vi "3.4.vi"() -> ()   [LabVIEW 2017]
panel:
  out "长度":dbl
  in  "字符串 2":string
  in  "字符串":string
  out "结果字符串":string
  in  "输入 1":dbl
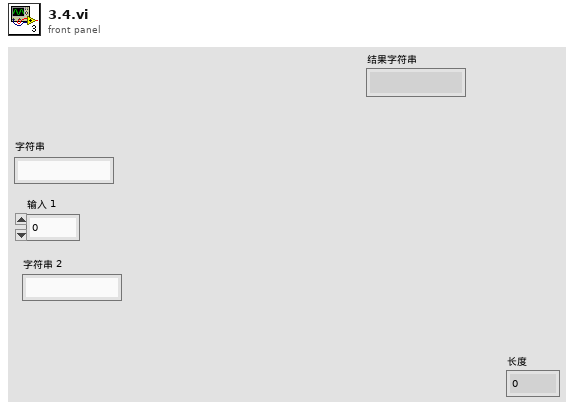
[diagram p1: front panel]
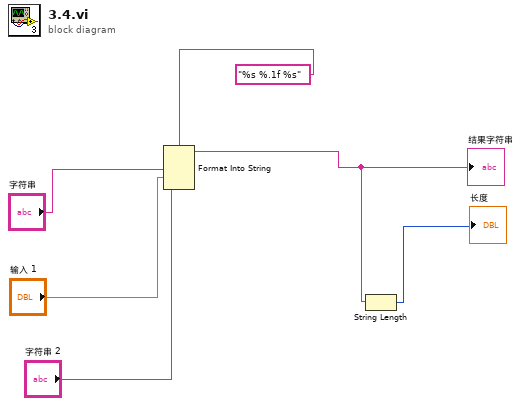
[diagram p0: block diagram]
diagram:
  n1 = Format Into String(format string="%s %.1f %s" ("格式字符串"), "字符串", "输入 1", "字符串 2") -> (resulting string=w2:string)  [unwired: 2 in, 1 out]
  "结果字符串" <- w2
  n2 = String Length(string=w2) -> (length=→"长度":i32)
